vi "analogSettings.vi"() -> ()   [LabVIEW 2020]
uses:
  <vilib>/Instr/_visa.llb/VISA Find Search Mode.ctl
  39ff5a11-8a08-4053-ac2d-0c6a76862e88.vi
  <userlib>/_OpenG.lib/array/array.llb/Filter 1D Array with Scalar (U16)__ogtk.vi
  SettingVariable.vi
  <resource>/objmgr/daqmx.rc
panel:
  in  "Cancel":bool
  in  "OK":bool
  out "Cancelled?":bool
  in  "电流源表2":u16(ring) caption="电流源表2：" items=["No Select COM", "ASRL1::INSTR", "ASRL2::INSTR", "ASRL10::INSTR"]
  in  "电流源表1":u16(ring) caption="电流源表1：" items=["No Select COM", "ASRL1::INSTR", "ASRL2::INSTR", "ASRL10::INSTR"]
  in  "串口电流值服务2":u16(ring) caption="串口电流值服务2：" items=["No Select COM", "ASRL1::INSTR", "ASRL2::INSTR", "ASRL10::INSTR"]
  in  "波特率":u32=57600 caption="波特率："
  in  "串口电流值服务1":u16(ring) caption="串口电流值服务1：" items=["No Select COM", "ASRL1::INSTR", "ASRL2::INSTR", "ASRL10::INSTR"]
  in  "电压脉冲开关":bool caption="电压脉冲开关："
  in  "电压脉冲卡选择":u16(ring) caption="电压脉冲卡选择：" items=["NI Simulated DAQ Device-0"]
  # "电压输出"
  # "电流源表"
  # "串口电流"
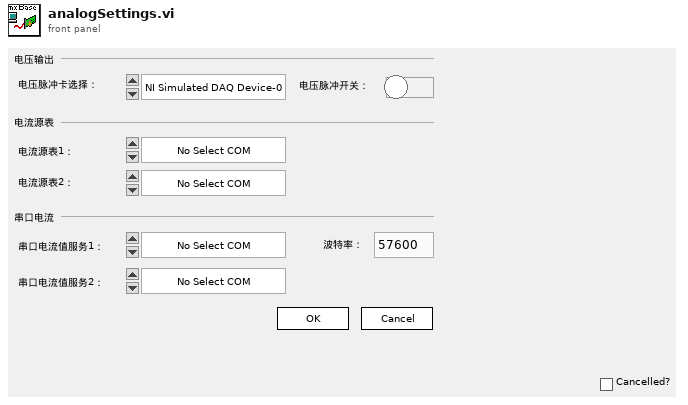
[diagram p1: front panel]
types:
  T1 = typedef "VISA Find Search Mode.ctl" = u32
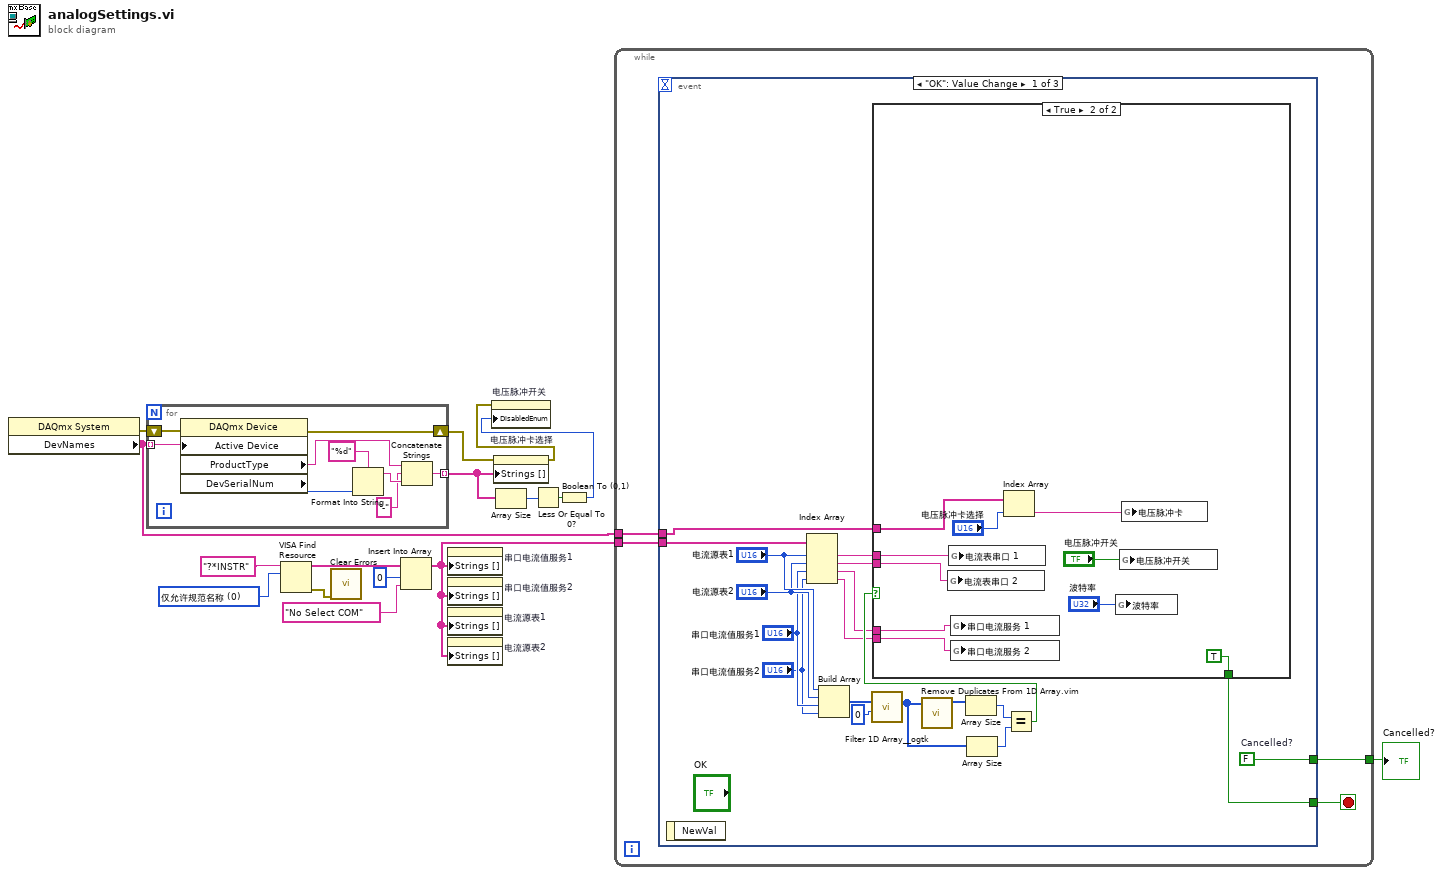
[diagram p0: block diagram]
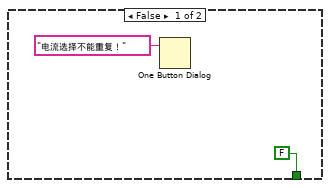
[diagram p2: hidden frame]
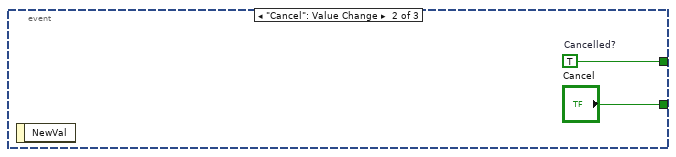
[diagram p3: hidden frame]
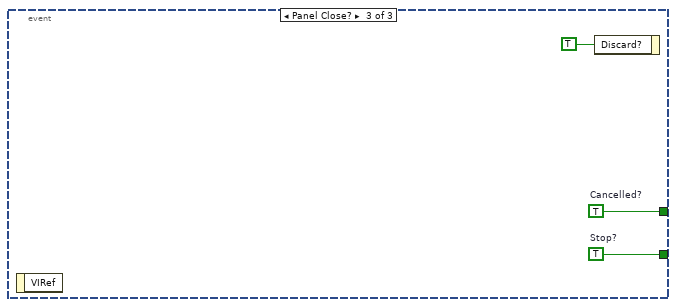
[diagram p4: hidden frame]
diagram:
  w13 = T1 0 items=["仅允许规范名称"=0, "只允许别名"=2, "包含匹配别名"=3, "包含所有别名"=4] ("Search Mode")
  n1 = property class="DAQmx System"() -> (error out=w6:errorcluster, "DevNames"=w1:tag[])  [unwired: 2 in, 1 out]
  n2 = for {
    tunnel: w1 -> [w25] mode=indexing
    tunnel: [w17] -> w5 mode=indexing
    shift-right: [w23] -> w2
    shift-left: w6 -> [w24]
    n3 = property class="DAQmx Device"(error in=w24, "Active Device"=w25) -> (error out=w23:errorcluster, "ProductType"=w20:string, "DevSerialNum"=w21:u32)  [unwired: 1 in, 1 out]
    n4 = Format Into String(format string="%d" ("格式字符串"), w21) -> (resulting string=w19:string)  [unwired: 2 in, 1 out]
    n5 = Concatenate Strings(w20, "-" ("字符串"), w19) -> (w17:string)
  }
  n6 = VISA Find Resource(10:w13, 11:"?*INSTR" ("表达式(\"?*\")")) -> (0:w14:errorcluster, 3:w11:string[])  [unwired: 1 in, 1 out]
  n7 = call <vilib>:"Clear Errors.vi"("error in (no error)"=w14) -> ()  [unwired: 5 in, 2 out]
  n8 = Insert Into Array(array=w11, index=0 ("索引"), new element="No Select COM" ("新元素/子数组")) -> (w3:string[])
  n9 = property on="串口电流值服务1" class="Ring (strict)"("Strings []"=w3) -> ()  [unwired: 2 in, 2 out]
  n10 = property on="串口电流值服务2" class="Ring (strict)"("Strings []"=w3) -> ()  [unwired: 2 in, 2 out]
  n11 = property on="电流源表1" class="Ring (strict)"("Strings []"=w3) -> ()  [unwired: 2 in, 2 out]
  n12 = property on="电流源表2" class="Ring (strict)"("Strings []"=w3) -> ()  [unwired: 2 in, 2 out]
  n13 = property on="电压脉冲卡选择" class="Ring (strict)"(error in=w2, "Strings []"=w5) -> (error out=w8:errorcluster)  [unwired: 1 in, 1 out]
  n14 = Array Size(array=w5) -> (size(s)=w10:i32)
  n15 = Less Or Equal To 0?(x=w10) -> (x <= 0?=w9:bool)
  n16 = Boolean To (0,1)(Boolean=w9) -> (0, 1=w7:i16)
  n17 = property on="电压脉冲开关" class="Bool (strict)"(error in=w8, "DisabledEnum"=w7) -> ()  [unwired: 1 in, 2 out]
  n18 = while {
    tunnel: [w28] -> w4
    tunnel: w3 -> [w27]
    tunnel: w1 -> [w26]
    stop <- w29 stop-if-true
    n19 = event shown="[0] \"OK\": Value Change" {
      selector: _ -> [_ _ _]
      dyn-events: _ -> [_ _ _]
      timeout: _ -> [_ _ _]
      tunnel: [w35 "Cancel" w64] -> w29
      tunnel: [w48 w62 w63] -> w28
      tunnel: w27 -> [w47 _ _]
      tunnel: w26 -> [w30 _ _]
      event "OK": Value Change {
        w48 = FALSE  # Cancelled?
        n20 = event-data() -> ()  [unwired: 1 in, 1 out]
        n21 = Index Array(array=w47, index #1="电流源表1", index #2="电流源表2", index #3="串口电流值服务1", index #4="串口电流值服务2") -> (element #1=w46:string, element #2=w45:string, element #3=w34:string, element #4=w33:string)
        n22 = Build Array("电流源表1", "电流源表2", "串口电流值服务1", "串口电流值服务2") -> (w42:u16[])
        n23 = call-poly <userlib>:"Filter 1D Array__ogtk.vi"("items to filter"=u16 0, "array"=w42) -> ("filtered array"=w39:u16[])  [unwired: 4 in, 1 out]
        n24 = call "Remove Duplicates From 1D Array.vim"("array"=w39) -> ("array with duplicates removed"=w40:u16[])  [unwired: 10 in]
        n25 = Array Size(array=w40) -> (size(s)=w38:i32)
        n26 = Array Size(array=w39) -> (size(s)=w37:i32)
        n27 = Equal?(x=w38, y=w37) -> (x = y?=w36:bool)
        n28 = case shown="True" w36 {
          tunnel: w46 -> [_ w60]
          tunnel: w34 -> [_ w59]
          tunnel: w33 -> [_ w58]
          tunnel: w45 -> [_ w57]
          tunnel: [FALSE ("Stop?") TRUE ("Stop?")] -> w35
          tunnel: w30 -> [_ w53]
          frame False {
            n29 = One Button Dialog(message="电流选择不能重复！") -> ()  [unwired: 1 in, 1 out]
          }
          frame True {
            n30 = global write "SettingVariable.vi" "电流表串口 2"(w57) -> ()
            n31 = global write "SettingVariable.vi" "电流表串口 1"(w60) -> ()
            n32 = global write "SettingVariable.vi" "串口电流服务 1"(w59) -> ()
            n33 = global write "SettingVariable.vi" "串口电流服务 2"(w58) -> ()
            n34 = Index Array(array=w53, index="电压脉冲卡选择") -> (element=w51:tag)
            n35 = global write "SettingVariable.vi" "波特率"("波特率") -> ()
            n36 = global write "SettingVariable.vi" "电压脉冲开关"("电压脉冲开关") -> ()
            n37 = global write "SettingVariable.vi" "电压脉冲卡"(w51) -> ()
          }
        }
      }
      event "Cancel": Value Change {
        w62 = TRUE  # Cancelled?
        n38 = event-data() -> ()  [unwired: 1 in, 1 out]
      }
      event Panel Close? {
        w63 = TRUE  # Cancelled?
        w64 = TRUE  # Stop?
        n39 = event-data() -> ()  [unwired: 1 in, 1 out]
        n40 = event-data("Discard?"=TRUE) -> ()  [unwired: 1 in, 1 out]
      }
    }
  }
  "Cancelled?" <- w4
